vi "Create DCM.vi"(6 "DCM Model":T1=enum."DCM-2301", 8 "error in (no error)":errorcluster, 11 "Section Ptr":T2 format="%.0x") -> (0 "error out":errorcluster, 3 "Section Ptr dup":T2 format="%.0x")   [LabVIEW 2016, in "DCM System Explorer.lvlib"]
uses:
  DCM System Explorer.lvlib
  <vilib>/NI Veristand/Custom Device API/Custom Device Item Ref.ctl
  Types/Bitfile Selection.ctl
  <vilib>/NI Veristand/Custom Device API/Custom Device Channel Type.ctl
  Shared/DCM Constants and GUIDs.vi
  <vilib>/NI VeriStand/Custom Device API/Custom Device API.lvlib
  DCM Shared.lvlib
  <vilib>/NI Veristand/Custom Device Tools/Custom Device Utility Library/Custom Device Utility Library.lvlib
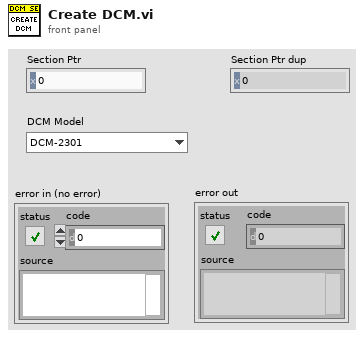
[diagram p1: front panel]
types:
  T1 = typedef "DCM System Explorer.lvlib/Bitfile Selection.ctl" = enum16{"Unknown (Disabled)", "DCM-2301", "DCM-2302", "DCM-2316", "DCM-2317"}
  T2 = typedef "Custom Device API.lvlib/Custom Device Item Ref.ctl" = u64
  T3 = typedef "Custom Device API.lvlib/Custom Device Channel Type.ctl" = enum16{"Input", "Output"}
  T4 = typedef "DCM Shared.lvlib/Channel.ctl" = cluster{"Name":string, "Units":string, "Default":dbl, "Description":string}
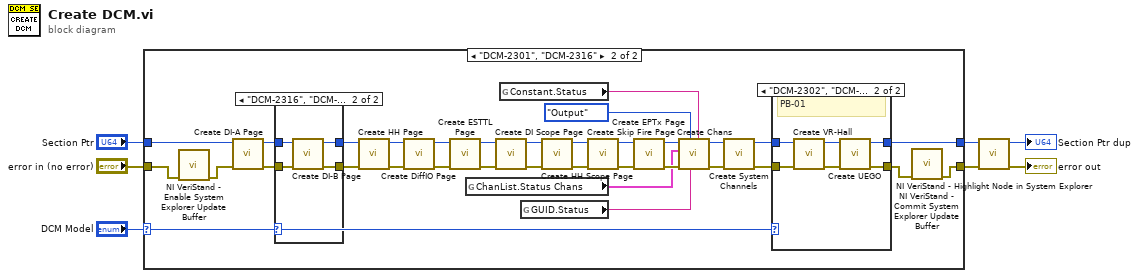
[diagram p0: block diagram]
diagram:
  n1 = case shown="\"DCM-2301\", \"DCM-2316\"" "DCM Model" {
    selector: "DCM Model" -> [_ w21]
    tunnel: "error in (no error)" -> [w8 w42]
    tunnel: "Section Ptr" -> [w9 w41]
    tunnel: [w8 w40] -> w5
    tunnel: [w9 w26] -> w6
    frame "Unknown (Disabled)", Default {
    }
    frame "DCM-2301", "DCM-2316" {
      n2 = call <vilib>:"NI VeriStand - Enable System Explorer Update Buffer.vi"("error in (no error)"=w42) -> ("error out"=w32:errorcluster)  [unwired: 10 in]
      n3 = call "Create DI-A Page.vi"("error in (no error)"=w32, "Section Ptr"=w41) -> ("error out"=w38:errorcluster, "Parent Ref out"=w39:T2)  [unwired: 8 in]
      n4 = case shown="\"DCM-2316\", \"DCM-2317\", Default" w21 {
        tunnel: w39 -> [w52 w56]
        tunnel: w38 -> [w51 w55]
        tunnel: [w51 w54] -> w36
        tunnel: [w52 w53] -> w35
        frame "DCM-2301", "DCM-2302" {
        }
        frame "DCM-2316", "DCM-2317", Default {
          n5 = call "Create DI-B Page.vi"("error in (no error)"=w55, "Section Ptr"=w56) -> ("error out"=w54:errorcluster, "Parent Ref out"=w53:T2)  [unwired: 8 in]
        }
      }
      n6 = call "Create HH Page.vi"("error in (no error)"=w36, "Section Ptr"=w35) -> ("error out"=w33:errorcluster, "Parent Ref out"=w34:T2)  [unwired: 8 in]
      n7 = call "Create DiffIO Page.vi"("error in (no error)"=w33, "Section Ptr"=w34) -> ("error out"=w18:errorcluster, "Parent Ref out"=w19:T2)  [unwired: 8 in]
      n8 = call "Create ESTTL Page.vi"("error in (no error)"=w18, "Section Ptr"=w19) -> ("error out"=w12:errorcluster, "Parent Ref out"=w13:T2)  [unwired: 8 in]
      n9 = global read "DCM Constants and GUIDs.vi" "ChanList.Status Chans"() -> (w24:T4[])
      n10 = call "Create DI Scope Page.vi"("error in (no error)"=w12, "Section Ptr"=w13) -> ("error out"=w20:errorcluster, "Parent Ref out"=w37:T2)  [unwired: 8 in]
      n11 = global read "DCM Constants and GUIDs.vi" "Constant.Status"() -> (w29:string)
      n12 = global read "DCM Constants and GUIDs.vi" "GUID.Status"() -> (w30:string)
      n13 = call "Create HH Scope Page.vi"("error in (no error)"=w20, "Section Ptr"=w37) -> ("error out"=w10:errorcluster, "Parent Ref out"=w11:T2)  [unwired: 8 in]
      n14 = call "Create Skip Fire Page.vi"("error in (no error)"=w10, "Section Ptr"=w11) -> ("error out"=w16:errorcluster, "Parent Ref out"=w17:T2)  [unwired: 8 in]
      n15 = call "Create EPTx Page.vi"("error in (no error)"=w16, "Section Ptr"=w17) -> ("error out"=w27:errorcluster, "Parent Ref out"=w28:T2)  [unwired: 8 in]
      n16 = call "Create Chans.vi"("New Section Name (none)"=w29, "new section GUID (\"\":del prot)"=w30, "Type"=Custom_Device_Channel_Type."Output", "error in (no error)"=w27, "Channels"=w24, "Section Ptr"=w28) -> ("error out"=w22:errorcluster, "Section Ptr dup"=w23:T2)  [unwired: 2 in, 2 out]
      n17 = call "Create System Channels.vi"("error in (no error)"=w22, "Parent Ref in"=w23) -> ("error out"=w14:errorcluster, "Parent Ref out"=w15:T2)  [unwired: 8 in]
      n18 = case shown="\"DCM-2302\", \"DCM-2317\"" w21 {
        tunnel: w15 -> [w44 w50]
        tunnel: [w44 w46] -> w26
        tunnel: [w43 w45] -> w25
        tunnel: w14 -> [w43 w48]
        frame "DCM-2301", "DCM-2316", Default {
          # "None"
        }
        frame "DCM-2302", "DCM-2317" {
          # "PB-01"
          n19 = call "Create VR-Hall.vi"("error in (no error)"=w48, "Parent Ref in"=w50) -> ("error out"=w47:errorcluster, "Parent Ref out"=w49:T2)  [unwired: 8 in]
          n20 = call "Create UEGO.vi"("error in (no error)"=w47, "Parent Ref in"=w49) -> ("error out"=w45:errorcluster, "Parent Ref out"=w46:T2)  [unwired: 8 in]
        }
      }
      n21 = call <vilib>:"NI VeriStand - Commit System Explorer Update Buffer.vi"("error in (no error)"=w25) -> ("error out"=w40:errorcluster)  [unwired: 10 in]
    }
  }
  n22 = call <vilib>:"NI VeriStand - Highlight Node in System Explorer.vi"("error in (no error)"=w5, "Item Ref in"=w6) -> ("error out"=→"error out":errorcluster, "Node Ptr dup"=→"Section Ptr dup":T2)  [unwired: 8 in]
